vi "Global_2.vi"() -> ()   [LabVIEW 2019]
panel:
  out "sampling rate":dbl
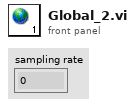
[diagram p1: front panel]
diagram:
